vi "Categorize Transaction.vi"(8 "error in (no error)":errorcluster, 9 "Transaction ID":string, 10 "Category ID":string, 11 "Budgetizer in":refnum<class "Budgetizer.lvclass">) -> (0 "error out":errorcluster, 3 "Budgetizer out":refnum<class "Budgetizer.lvclass">)   [LabVIEW 2018, in "Budgetizer.lvclass"]
uses:
  Budgetizer.lvclass
  Budgetizer.lvclass/Budgetizer.ctl
  database/Database.lvclass
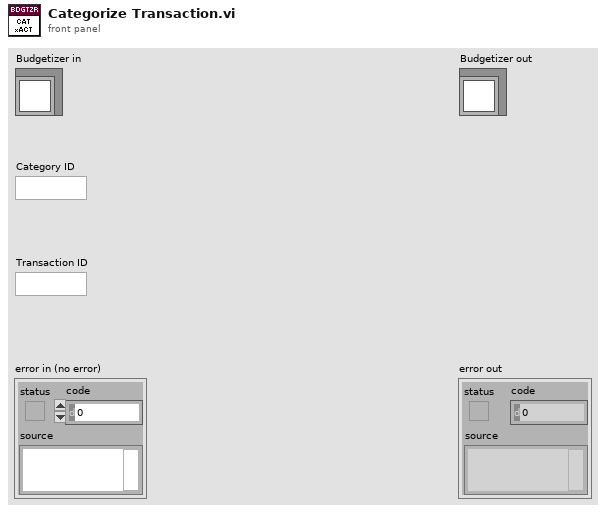
[diagram p1: front panel]
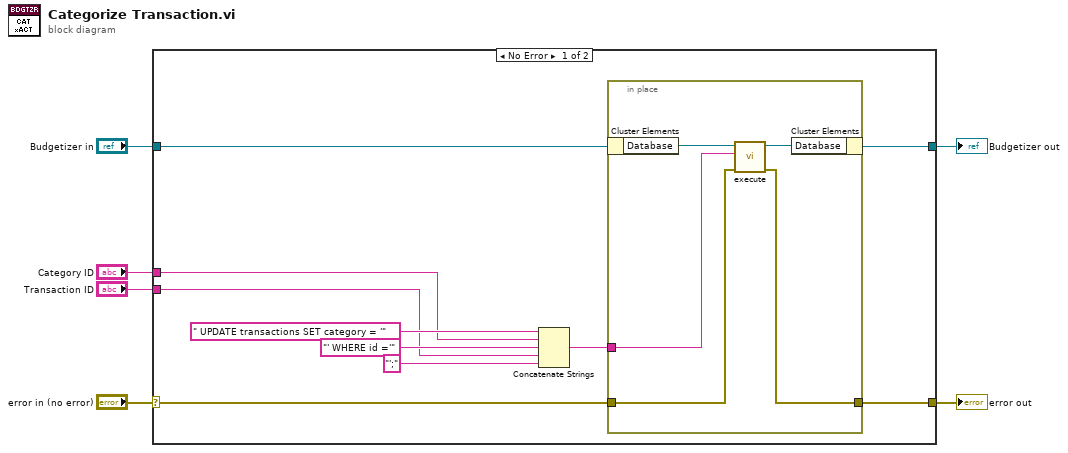
[diagram p0: block diagram]
diagram:
  n1 = case shown="No Error" "error in (no error)" {
    selector: "error in (no error)" -> [w9 w23]
    tunnel: [w8 w23] -> w5
    tunnel: [w10 w22] -> w3
    tunnel: "Budgetizer in" -> [w11 w22]
    tunnel: "Transaction ID" -> [w12 _]
    tunnel: "Category ID" -> [w15 _]
    frame No Error {
      n2 = Concatenate Strings(" UPDATE transactions SET category = '", w15, "' WHERE id ='", w12, "';") -> (w7:string)
      n3 = in-place {
        in-place-border: w9 -> [w19]
        in-place-border: [w18] -> w8
        in-place-border: w7 -> [w17]
        n4 = in-place-cluster #1(w11) -> ("Database"=w21:refnum<class "Database.lvclass">)
        n5 = call "execute.vi"("error in (no error)"=w19, "SQL query"=w17, "Database in"=w21) -> ("error out"=w18:errorcluster, "Database out"=w20:refnum<class "Database.lvclass">)  [unwired: 7 in]
        n6 = in-place-cluster #1("Database"=w20) -> (w10:refnum<class "Budgetizer.lvclass">)
      }
    }
    frame Error {
    }
  }
  "error out" <- w5
  "Budgetizer out" <- w3
